vi "GetSensorValues.vi"(1 "Ref_BuiltInAccelerometer":T8={"DevStatus"={"status"=FALSE, "code"=0, "source"=""}, "Scaling"={"Gain (VoltsPerG)"=0.0, "Center Voltage"=0.0}, "Analog Channels"={"X-Axis"=enum."Invalid", "Y-Axis"=enum."Invalid", "Z-Axis"=enum."Invalid"}, "I2C Bus"=enum."Invalid", "SPI Bus"=enum."Invalid", "Accel Range"=0, "ADXL Axes"={"X-Axis"=FALSE, "Y-Axis"=FALSE, "Z-Axis"=FALSE}, "Handle"=0, "Device Address"=0, "Accel Type"=enum."Analog"} {"Device Address" format="%.0x"; "Accel Range" items=["+/- 2 g", "+/- 4 g", "+/- 8 g", "+/- 16 g"]}, 3 "Rear Prox Sensor":T6, 4 "Right Prox Sensor":T6, 5 "Left Prox Sensor":T6, 6 "Upper Pressure Transducer":T6, 8 "Ref_Compressor":T15, 9 "Front-Right Prox Sensor":T6, 10 "Ref_ElevatorEncoder":T1={"DeviceStatus"={"status"=FALSE, "code"=0, "source"=""}, "Type"=enum."PWM", "PWM"={"PWM Channel"=enum."Invalid", "DeadBand"={"Name"="", "maxPositivePwm"=0, "minPositivePwm"=0, "centerPwm"=0, "maxNegativePwm"=0, "minNegativePwm"=0, "angularRange"=0}}, "CAN"={"Device Number"=0, "SetOutput VI Ref"=variant, "GetOutput VI Ref"=variant, "Enable VI Ref"=variant, "Disable VI Ref"=variant, "Data"=variant}, "Invert"=FALSE, "DIO PWM"={"PWM \"Enable\" Channel"=enum."Invalid", "DIOChannel"=enum."Invalid", "PWM Rate"=0.0}}, 11 "Front-Left Prox Sensor":T6, 12 "Ref_ElevatorLimitSwitches":T1={"DeviceStatus"={"status"=FALSE, "code"=0, "source"=""}, "Type"=enum."PWM", "PWM"={"PWM Channel"=enum."Invalid", "DeadBand"={"Name"="", "maxPositivePwm"=0, "minPositivePwm"=0, "centerPwm"=0, "maxNegativePwm"=0, "minNegativePwm"=0, "angularRange"=0}}, "CAN"={"Device Number"=0, "SetOutput VI Ref"=variant, "GetOutput VI Ref"=variant, "Enable VI Ref"=variant, "Disable VI Ref"=variant, "Data"=variant}, "Invert"=FALSE, "DIO PWM"={"PWM \"Enable\" Channel"=enum."Invalid", "DIOChannel"=enum."Invalid", "PWM Rate"=0.0}}, 15 "Tank Pressure Transducer":T6, 19 "Ground Prox Sensor":T6, 20 "Ref_Drive 1R":T1, 21 "Ref_Drive 2R":T1, 22 "Ref_Drive 3L":T1, 23 "Ref_Drive 4L":T1, 24 "Ref_Drive 5L":T1, 26 "Ref_Drive 6R":T1) -> ()   [LabVIEW 2018]
uses:
  <vilib>/Rock Robotics/WPI/AnalogChannel/WPI_AnalogChannelDevRef.ctl
  <vilib>/Rock Robotics/SystemInterfaces/AI/FPGA_AIChannel.ctl
  <vilib>/Rock Robotics/WPI/Compressor/WPI_CompressorDevRef.ctl
  <vilib>/Rock Robotics/WPI/MotorControl/WPI_MotorControlDeviceRef.ctl
  <vilib>/Rock Robotics/WPI/MotorControl/WPI_MotorControlType.ctl
  <vilib>/Rock Robotics/SystemInterfaces/DIO/FPGA_DIOPWMChannel.ctl
  <vilib>/Rock Robotics/WPI/PWM/WPI_PWMDeadband.ctl
  <vilib>/Rock Robotics/SystemInterfaces/DIO/FPGA_DIOChannel.ctl
  <vilib>/Rock Robotics/WPI/Accelerometer/WPI_AccelerometerDevRef.ctl
  <vilib>/Rock Robotics/WPI/Accelerometer/WPI_AccelerometerScaling.ctl
  <vilib>/Rock Robotics/WPI/Accelerometer/WPI_AccelerometerAnalogChannels.ctl
  <vilib>/Rock Robotics/SystemInterfaces/i2clib/i2c_bus.ctl
  <vilib>/Rock Robotics/SystemInterfaces/spilib/spi_bus.ctl
  <vilib>/Rock Robotics/WPI/Accelerometer/ADXL345 Range.ctl
  <vilib>/Rock Robotics/WPI/Accelerometer/WPI_AccelerometerADXL345 Axes.ctl
  <vilib>/Rock Robotics/WPI/DriverStation/WPI_DriverStationRobotMode2.ctl
  <vilib>/Analysis/baseanly.llb/Mean (DBL).vi
  SensorReadings.vi
  RefNums_Actuators.vi
  RobotStates.vi
  Inputs_DriverStation.vi
  <vilib>/Rock Robotics/WPI/ThirdParty/Phoenix-LabVIEW/Motor Controller/Get/CTRE_Phoenix_MotorController_GetLimitSwitchStates.vi
  <vilib>/Rock Robotics/WPI/ThirdParty/Phoenix-LabVIEW/Motor Controller/Get/CTRE_Phoenix_MotorController_GetSelectedSensorData.vi
  <vilib>/gmath/NI_Gmath.lvlib
  <vilib>/Analysis/NI_AALBase.lvlib
  <vilib>/Analysis/NI_AALPro.lvlib
panel:
  out "Pressure Leak (psi/min)":dbl format="%#_3f"
  in  "Normal Elevator Std (A)":dbl=35.0
  in  "Off Ground Time (ms)":u32=100
  in  "On Ground Time (ms)":u32=1000
  in  "Ground Distance (in)":dbl=6.0
  in  "Plot Drive Encoder Data":bool
  in  "Tank Pressure Voltage Table":dbl[](array[numeric])=[0.4, 0.7, 0.9, 1.2, 1.4, 1.7, 1.9, 2.3, 2.5, 2.8, 3.0, 3.3] format="%_6g"
  in  "Tank Pressure PSI Table":dbl[](array[numeric])=[0.0, 10.0, 20.0, 30.0, 40.0, 50.0, 60.0, 70.0, 80.0, 90.0, 100.0, 115.0] format="%_6g"
  in  "LR Voltage Table":dbl[](array[numeric])=[0.43, 0.45, 0.47, 0.55, 0.6, 0.68, 0.72, 0.81, 0.86, 0.98, 1.13, 1.36, 1.53, 1.77, 1.99, 2.26, 2.52, 2.76] format="%_6g"
  in  "LR Distance Table":dbl[](array[numeric])=[150.661, 140.6, 133.7, 120.9, 110.1, 95.3, 90.1, 80.0, 73.7, 64.6, 55.9, 45.6, 40.2, 35.0, 29.6, 24.3, 19.6, 14.8] format="%_6g"
  in  "Suction Threshold (V)":dbl=0.1
  in  "SR Voltage Table":dbl[](array[numeric])=[3.15, 2.82, 2.51, 2.16, 1.92, 1.7, 1.49, 1.3, 1.12, 0.97, 0.87, 0.79, 0.72, 0.64, 0.61, 0.58, 0.52, 0.47, 0.46, 0.45, 0.43, 0.41] format="%_6g"
  in  "SR Distance Table":dbl[](array[numeric])=[4.6, 6.6, 8.3, 10.4, 12.2, 14.1, 16.5, 19.9, 23.6, 28.2, 32.6, 36.8, 40.9, 46.3, 49.9, 53.7, 58.3, 63.5, 67.5, 71.5, 75.1, 78.9] format="%_6g"
  out "Drive Encoder Velocities":cluster{dbl, dbl}(graph)
  # "*** Alpha was set to 6 inches ***"
  # "*** Beta was set to 12 inches ***"
  # "ADXL"
  # "Analog"
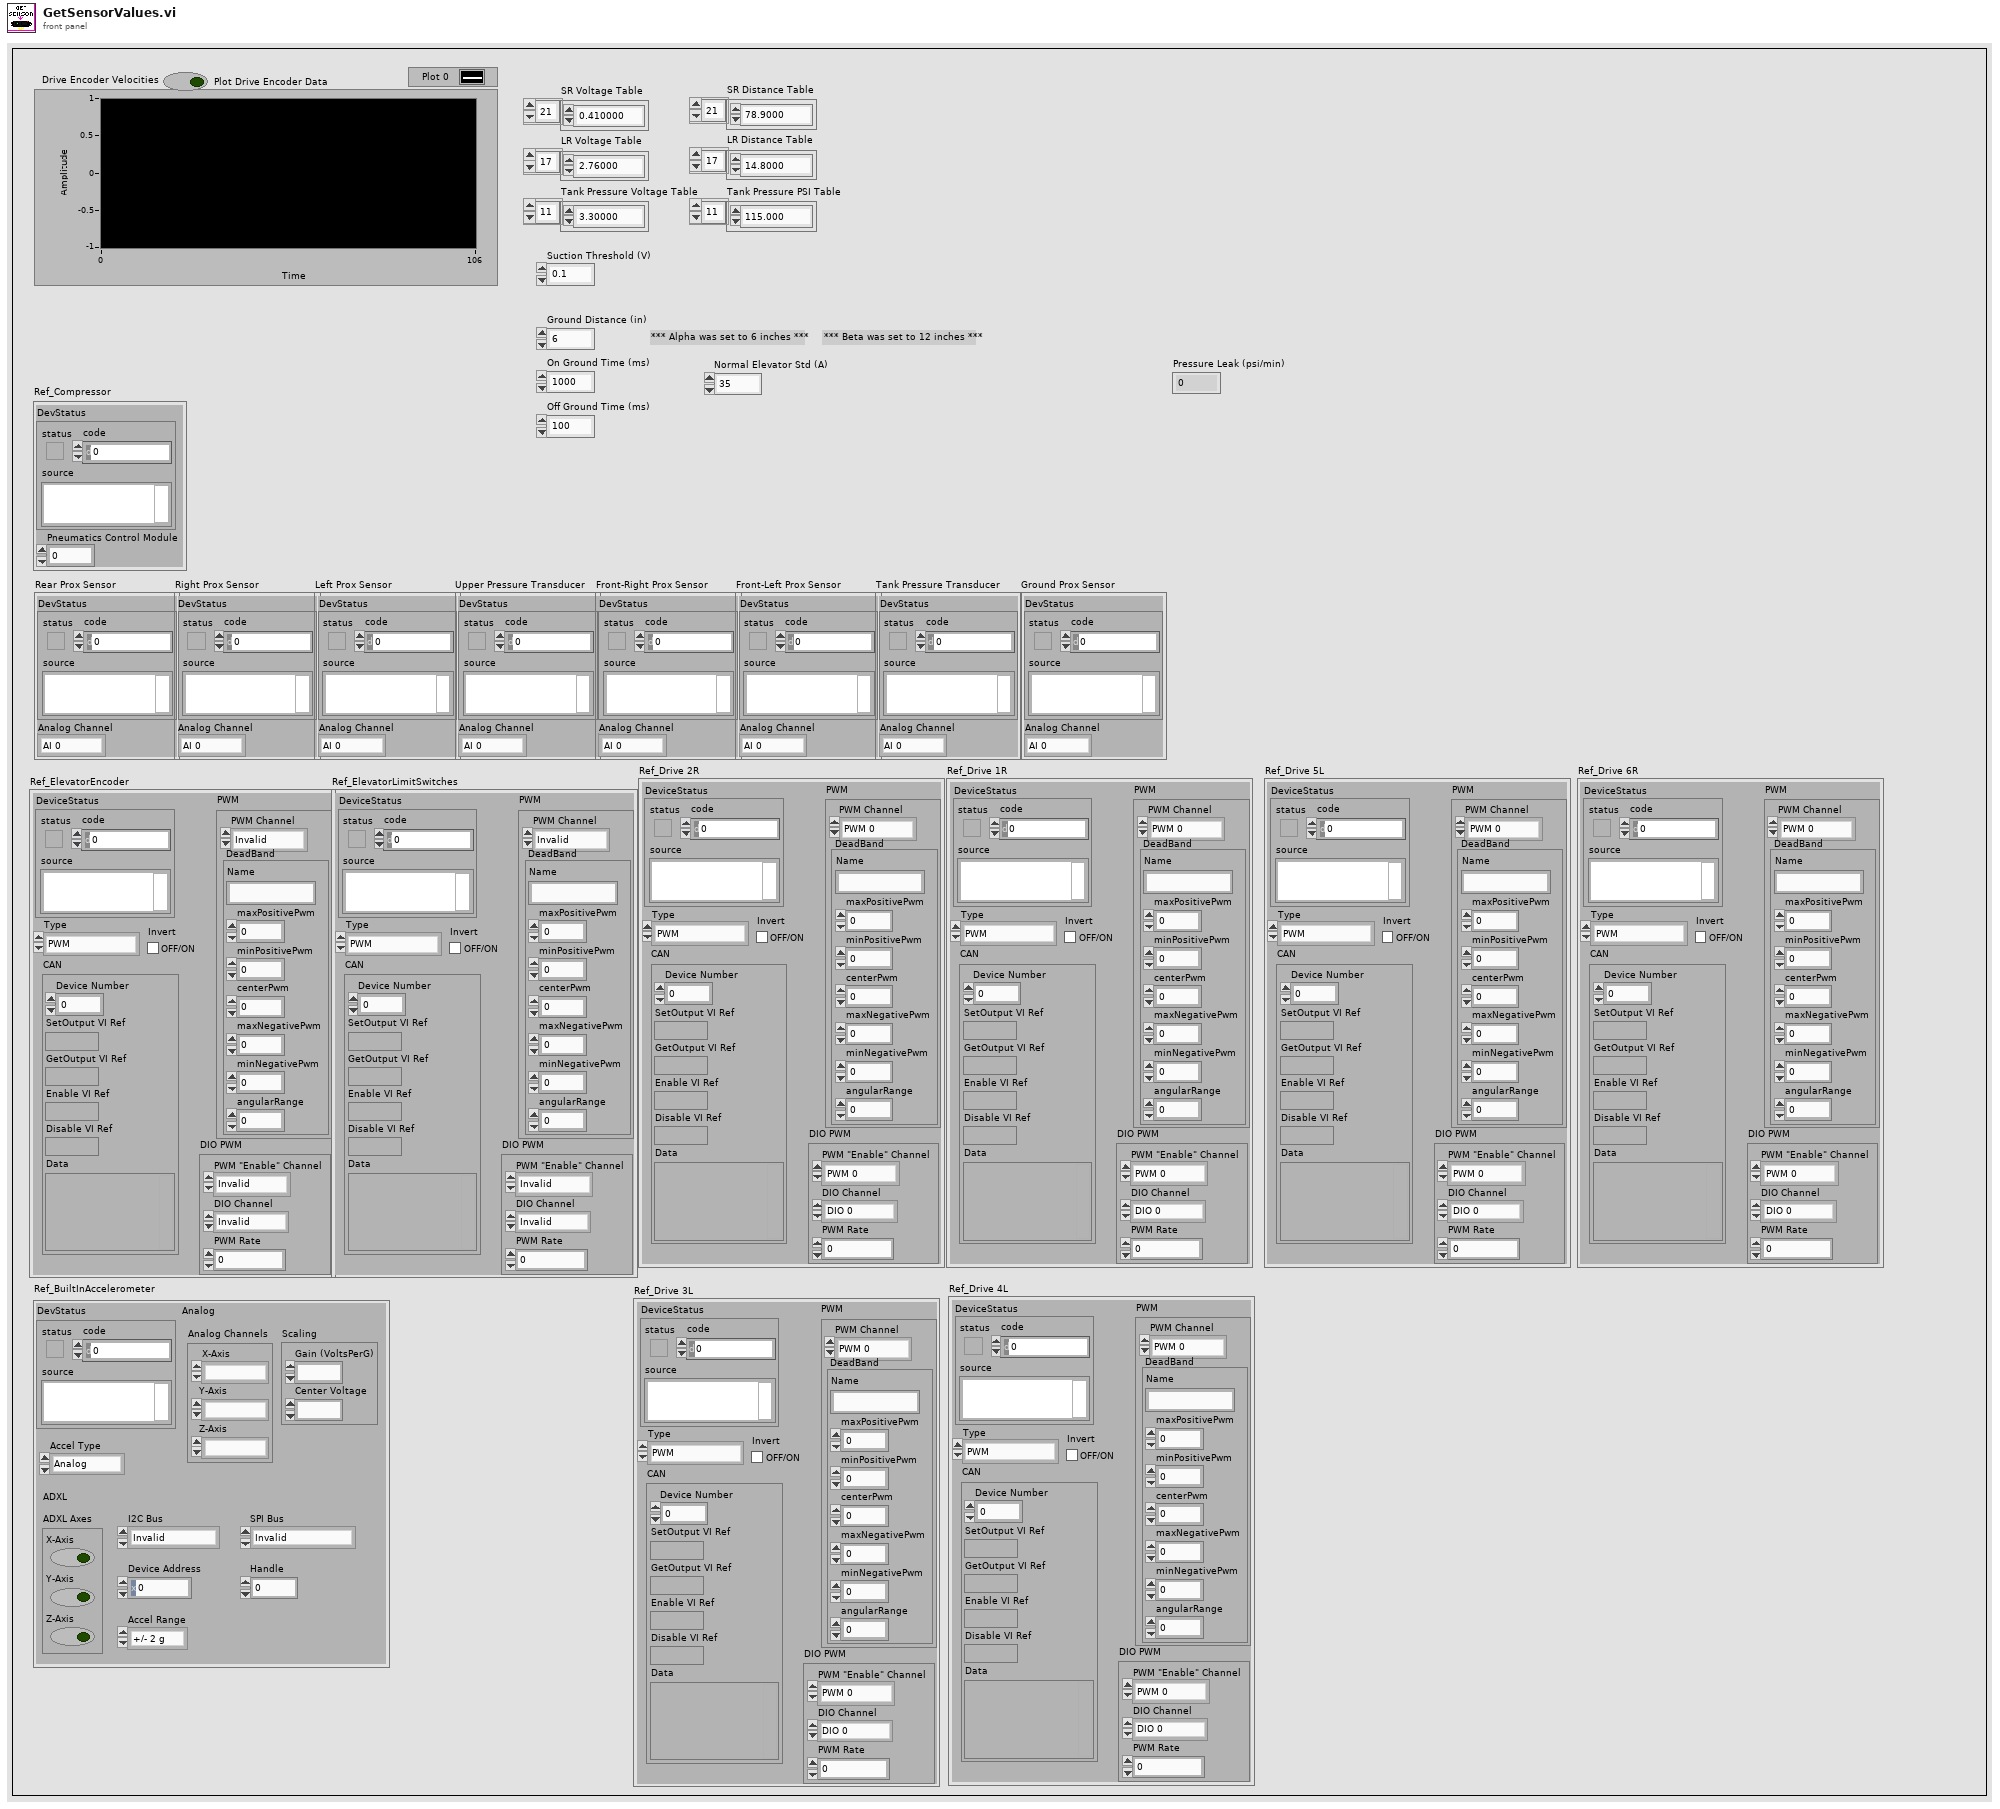
[diagram p1: front panel]
types:
  T1 = typedef "WPI_MotorControlDeviceRef.ctl" = cluster{"DeviceStatus":errorcluster, "Type":T2, "PWM":cluster{"PWM Channel":T3, "DeadBand":T4}, "CAN":cluster{"Device Number":u8, "SetOutput VI Ref":variant, "GetOutput VI Ref":variant, "Enable VI Ref":variant, "Disable VI Ref":variant, "Data":variant}, "Invert":bool, "DIO PWM":cluster{"PWM \"Enable\" Channel":T3, "DIOChannel":T5, "PWM Rate":dbl}}
  T2 = typedef "WPI_MotorControlType.ctl" = enum16{"PWM", "CAN", "DIO PWM"}
  T3 = typedef "FPGA_DIOPWMChannel.ctl" = enum8{"PWM 0", "PWM 1", "PWM 2", "PWM 3", "PWM 4", "PWM 5", "PWM 6", "PWM 7", "PWM 8", "PWM 9", "PWM MXP 0", "PWM MXP 1", "PWM MXP 2", "PWM MXP 3", "PWM MXP 4", "PWM MXP 5", "PWM MXP 6", "PWM MXP 7", "PWM MXP 8", "PWM MXP 9", "Invalid"}
  T4 = typedef "WPI_PWMDeadband.ctl" = cluster{"Name":string, "maxPositivePwm":i32, "minPositivePwm":i32, "centerPwm":i32, "maxNegativePwm":i32, "minNegativePwm":i32, "angularRange":u16}
  T5 = typedef "FPGA_DIOChannel.ctl" = enum8{"DIO 0", "DIO 1", "DIO 2", "DIO 3", "DIO 4", "DIO 5", "DIO 6", "DIO 7", "DIO 8", "DIO 9", "DIO MXP 0", "DIO MXP 1", "DIO MXP 2", "DIO MXP 3", "DIO MXP 4", "DIO MXP 5", "DIO MXP 6", "DIO MXP 7", "DIO MXP 8", "DIO MXP 9", "DIO MXP 10", "DIO MXP 11", "DIO MXP 12", "DIO MXP 13", "DIO MXP 14", "DIO MXP 15", "SPI Port CS1", "SPI Port CS2", "SPI Port CS3", "SPI Port MISO", "SPI Port MOSI", "Invalid"}
  T6 = typedef "WPI_AnalogChannelDevRef.ctl" = cluster{"DevStatus":errorcluster, "Analog Channel":T7}
  T7 = typedef "FPGA_AIChannel.ctl" = enum8{"AI 0", "AI 1", "AI 2", "AI 3", "AI MXP 0", "AI MXP 1", "AI MXP 2", "AI MXP 3", "Invalid"}
  T8 = typedef "WPI_AccelerometerDevRef.ctl" = cluster{"DevStatus":errorcluster, "Scaling":T9, "Analog Channels":T10, "I2C Bus":T11, "SPI Bus":T12, "Accel Range":T13, "ADXL Axes":T14, "Handle":i32, "Device Address":u8, "Accel Type":enum16{"Analog", "ADXL345 I2C", "ADXL345 SPI", "Internal", "ADXL362 SPI"}}
  T9 = typedef "WPI_AccelerometerScaling.ctl" = cluster{"Gain (VoltsPerG)":dbl, "Center Voltage":dbl}
  T10 = typedef "WPI_AccelerometerAnalogChannels.ctl" = cluster{"X-Axis":T7, "Y-Axis":T7, "Z-Axis":T7}
  T11 = typedef "i2c_bus.ctl" = enum16{"I2C On-Board", "I2C MXP", "Invalid"}
  T12 = typedef "spi_bus.ctl" = enum16{"SPI On-Board, CS0", "SPI On-Board, CS1", "SPI On-Board, CS2", "SPI On-Board, CS3", "SPI MXP", "Invalid"}
  T13 = typedef "ADXL345 Range.ctl" = u8
  T14 = typedef "WPI_AccelerometerADXL345 Axes.ctl" = cluster{"X-Axis":bool, "Y-Axis":bool, "Z-Axis":bool}
  T15 = typedef "WPI_CompressorDevRef.ctl" = cluster{"DevStatus":errorcluster, "Pneumatics Control Module":u8}
  T16 = typedef "WPI_DriverStationRobotMode2.ctl" = enum16{"Autonomous Disabled", "Autonomous Enabled", "Teleop Disabled", "Teleop Enabled", "Disconnected", "Finish", "Test Disabled", "Test Enabled", "Emergency Stopped"}
  T17 = cluster{"X-Axis":dbl, "Y-Axis":dbl, "Z-Axis":dbl}
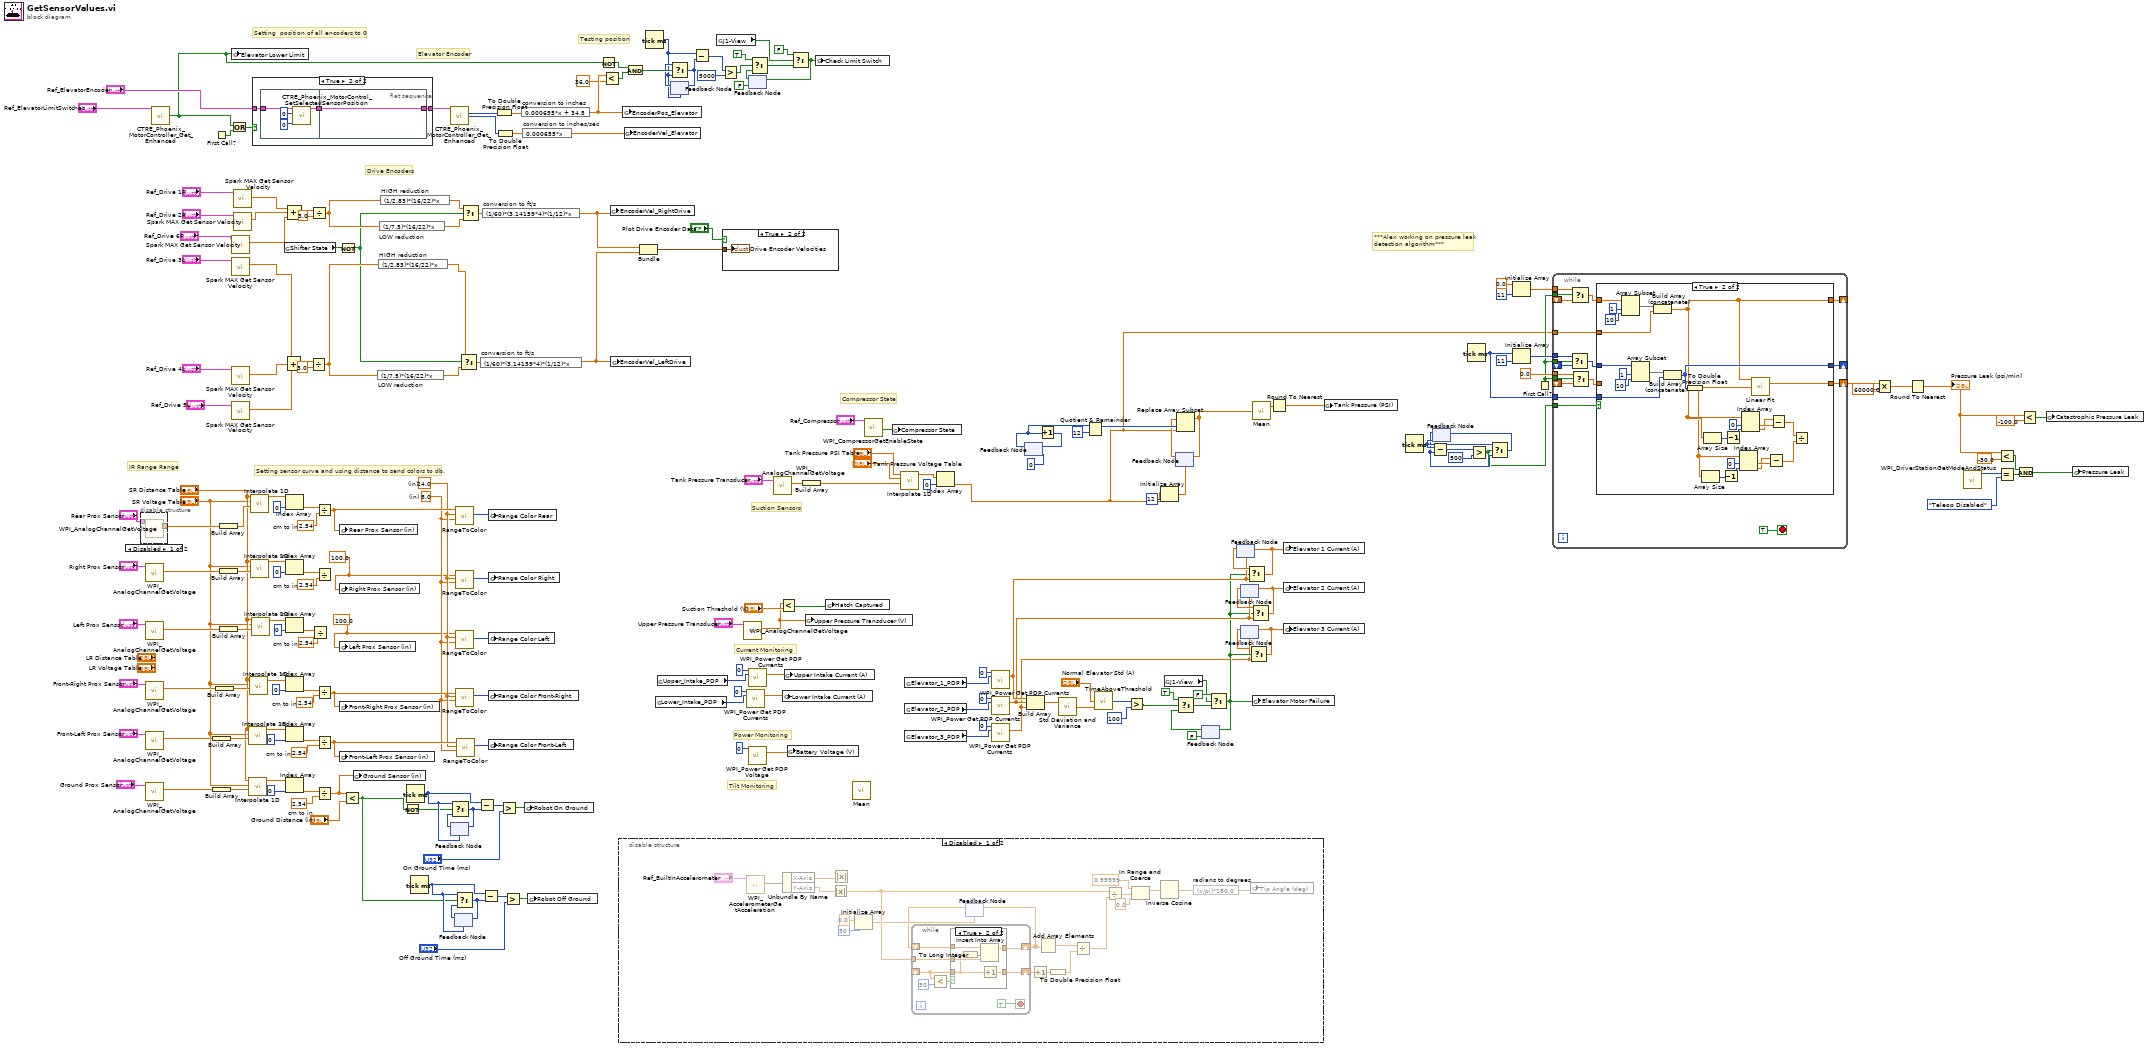
[diagram p0: block diagram]
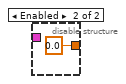
[diagram p3: hidden frame]
diagram:
  w50 = 100.0
  w51 = 100.0
  w121 = 2.54  # cm to in
  w177 = 2.54  # cm to in
  w170 = 8.0  # (in)
  w171 = 24.0  # (in)
  w194 = 2.54  # cm to in
  w200 = 2.54  # cm to in
  w207 = 2.54  # cm to in
  w214 = 2.54  # cm to in
  # "***Alex working on pressure leak\ndetection algorithm***"
  # "Elevator Encoder"
  # "Tilt Monitoring"
  # "Drive Encoders"
  # "Power Monitoring"
  # "Testing position"
  # "Setting  position of all encoders to 0"
  # "Setting sensor curve and using distance to send colors to db."
  # "Current Monitoring"
  # "Suction Sensors"
  # "Compressor State"
  # "IR Range Range"
  n1 = disable-structure shown="Disabled" {
    disable-tunnel: [w220 0.0 ("Voltage")] -> w218
    disable-tunnel: "Rear Prox Sensor" -> [w219 _]
    frame Disabled {
      n2 = call <vilib>:"WPI_AnalogChannelGetVoltage.vi"("AIDeviceRef"=w219) -> ("Voltage"=w220:dbl)  [unwired: 8 in, 2 out]
    }
    frame Enabled {
    }
  }
  n3 = call <vilib>:"WPI_AnalogChannelGetVoltage.vi"("AIDeviceRef"="Right Prox Sensor") -> ("Voltage"=w212:dbl)  [unwired: 8 in, 2 out]
  n4 = call <vilib>:"WPI_AnalogChannelGetVoltage.vi"("AIDeviceRef"="Left Prox Sensor") -> ("Voltage"=w205:dbl)  [unwired: 8 in, 2 out]
  n5 = call <vilib>:"WPI_AnalogChannelGetVoltage.vi"("AIDeviceRef"="Front-Right Prox Sensor") -> ("Voltage"=w182:dbl)  [unwired: 8 in, 2 out]
  n6 = call <vilib>:"WPI_AnalogChannelGetVoltage.vi"("AIDeviceRef"="Front-Left Prox Sensor") -> ("Voltage"=w175:dbl)  [unwired: 8 in, 2 out]
  n7 = call <vilib>:"WPI_AnalogChannelGetVoltage.vi"("AIDeviceRef"="Ground Prox Sensor") -> ("Voltage"=w120:dbl)  [unwired: 8 in, 2 out]
  n8 = call-poly <vilib>:"CTRE_Phoenix_MotorController_Get_Enhanced.vi"("PhoenixMotorControlDevRef"="Ref_ElevatorLimitSwitches") -> ("Reverse Limit Closed?"=w67:bool)  [unwired: 11 in, 3 out]
  n9 = First Call?() -> (First Call?: T/F=w125:bool)
  n10 = Build Array(w175) -> (w180:dbl[])
  n11 = Build Array(w120) -> (w124:dbl[])
  n12 = Build Array(w182) -> (w198:dbl[])
  n13 = Build Array(w218) -> (w192:dbl[])
  n14 = Build Array(w212) -> (w211:dbl[])
  n15 = Build Array(w205) -> (w204:dbl[])
  n16 = Or(x=w67, y=w125) -> (x .or. y?=w126:bool)
  n17 = global write "SensorReadings.vi" "Elevator Lower Limit"(w67) -> ()
  n18 = call <vilib>:"Spark MAX Get Sensor Velocity.vi"("MotorControlDevRef in"="Ref_Drive 6R") -> ("Sensor Velocity"=w47:dbl)  [unwired: 7 in, 3 out]
  n19 = call <vilib>:"Spark MAX Get Sensor Velocity.vi"("MotorControlDevRef in"="Ref_Drive 3L") -> ("Sensor Velocity"=w153:dbl)  [unwired: 7 in, 3 out]
  n20 = call <vilib>:"Spark MAX Get Sensor Velocity.vi"("MotorControlDevRef in"="Ref_Drive 4L") -> ("Sensor Velocity"=w152:dbl)  [unwired: 7 in, 3 out]
  n21 = call <vilib>:"Spark MAX Get Sensor Velocity.vi"("MotorControlDevRef in"="Ref_Drive 5L") -> ("Sensor Velocity"=w46:dbl)  [unwired: 7 in, 3 out]
  n22 = call <vilib>:"Spark MAX Get Sensor Velocity.vi"("MotorControlDevRef in"="Ref_Drive 1R") -> ("Sensor Velocity"=w158:dbl)  [unwired: 7 in, 3 out]
  n23 = call <vilib>:"Spark MAX Get Sensor Velocity.vi"("MotorControlDevRef in"="Ref_Drive 2R") -> ("Sensor Velocity"=w99:dbl)  [unwired: 7 in, 3 out]
  n24 = call <vilib>:"Interpolate 1D.vi"("xi"=w180, "X"="SR Voltage Table", "Y"="SR Distance Table") -> ("yi"=w174:dbl[])  [unwired: 6 in, 2 out]
  n25 = call <vilib>:"Interpolate 1D.vi"("xi"=w124, "X"="SR Voltage Table", "Y"="SR Distance Table") -> ("yi"=w119:dbl[])  [unwired: 6 in, 2 out]
  n26 = call <vilib>:"Interpolate 1D.vi"("xi"=w198, "X"="SR Voltage Table", "Y"="SR Distance Table") -> ("yi"=w195:dbl[])  [unwired: 6 in, 2 out]
  n27 = call <vilib>:"Interpolate 1D.vi"("xi"=w192, "X"="SR Voltage Table", "Y"="SR Distance Table") -> ("yi"=w215:dbl[])  [unwired: 6 in, 2 out]
  n28 = call <vilib>:"Interpolate 1D.vi"("xi"=w211, "X"="SR Voltage Table", "Y"="SR Distance Table") -> ("yi"=w208:dbl[])  [unwired: 6 in, 2 out]
  n29 = call <vilib>:"Interpolate 1D.vi"("xi"=w204, "X"="SR Voltage Table", "Y"="SR Distance Table") -> ("yi"=w201:dbl[])  [unwired: 6 in, 2 out]
  n30 = case shown="True" w126 {
    tunnel: "Ref_ElevatorEncoder" -> [w222 w225]
    tunnel: [w222 w223] -> w131
    frame False {
    }
    frame True {
      n31 = flat-sequence {
        tunnel: w225 -> [w229]
        tunnel: [w228] -> w224
        tunnel: [w230] -> w223
        tunnel: w224 -> [w230]
        frame #0 {
          n32 = call <vilib>:"CTRE_Phoenix_MotorControl_SetSelectedSensorPosition.vi"("pidLoopIdx"=u32 0, "New Sensor Position"=0, "PhoenixMotorControlDevRef"=w229) -> ("PhoenixMotorControlDevRef"=w228:T1)  [unwired: 7 in, 1 out]
        }
        frame #1 {
        }
      }
    }
  }
  n33 = global read "RobotStates.vi" "Shifter State"() -> (w145:bool)
  n34 = Index Array(array=w215, index=0) -> (element=w216:dbl)
  n35 = Index Array(array=w208, index=0) -> (element=w209:dbl)
  n36 = Index Array(array=w201, index=0) -> (element=w202:dbl)
  n37 = Index Array(array=w195, index=0) -> (element=w196:dbl)
  n38 = Index Array(array=w174, index=0) -> (element=w178:dbl)
  n39 = Index Array(array=w119, index=0) -> (element=w122:dbl)
  n40 = Compound Arithmetic op=ADD(w153, w152, w46) -> (w155:dbl)
  n41 = Compound Arithmetic op=ADD(w158, w99, w47) -> (w157:dbl)
  n42 = Divide(x=w155, y=3.0) -> (x/y=w146:dbl)
  n43 = Divide(x=w157, y=3.0) -> (x/y=w149:dbl)
  n44 = Divide(x=w202, y=w200) -> ()  [unwired: 1 out]
  n45 = Divide(x=w216, y=w214) -> (x/y=w191:dbl)
  n46 = Divide(x=w209, y=w207) -> ()  [unwired: 1 out]
  n47 = Divide(x=w196, y=w194) -> (x/y=w190:dbl)
  n48 = Divide(x=w178, y=w177) -> (x/y=w176:dbl)
  n49 = Divide(x=w122, y=w121) -> (x/y=w102:dbl)
  n50 = Not(x=w145) -> (.not. x?=w133:bool)
  n51 = global write "SensorReadings.vi" "Rear Prox Sensor (in)"(w191) -> ()
  n52 = global write "SensorReadings.vi" "Right Prox Sensor (in)"(w51) -> ()
  n53 = global write "SensorReadings.vi" "Left Prox Sensor (in)"(w50) -> ()
  n54 = global write "SensorReadings.vi" "Front-Right Prox Sensor (in)"(w190) -> ()
  n55 = global write "SensorReadings.vi" "Front-Left Prox Sensor (in)"(w176) -> ()
  n56 = Less?(x=w102, y="Ground Distance (in)") -> (x < y?=w101:bool)
  n57 = global write "SensorReadings.vi" "Ground Sensor (in)"(w102) -> ()
  n58 = expression code="(1/7.5)*(16/22)*x" "LOW reduction"(w146) -> (w147:dbl)
  n59 = expression code="(1/2.83)*(16/22)*x" "HIGH reduction"(w146) -> (w148:dbl)
  n60 = expression code="(1/7.5)*(16/22)*x" "LOW reduction"(w149) -> (w150:dbl)
  n61 = expression code="(1/2.83)*(16/22)*x" "HIGH reduction"(w149) -> (w151:dbl)
  n62 = Not(x=w101) -> (.not. x?=w100:bool)
  n63 = Tick Count (ms)() -> (millisecond timer value=w112:u32)
  n64 = Tick Count (ms)() -> (millisecond timer value=w107:u32)
  n65 = feedback #1(w112) -> (w114:u32)
  n66 = call-poly <vilib>:"CTRE_Phoenix_MotorController_Get_Enhanced.vi"("PhoenixMotorControlDevRef"=w131) -> ("Position (Raw Sensor Units)"=w130:i32, "Velocity (Raw Sensor Units per 100 ms)"=w128:i32)  [unwired: 11 in, 2 out]
  n67 = Select(t=w112, s=w100, f=w114) -> (s? t:f=w113:u32)
  n68 = feedback-in #1(w113) -> ()
  n69 = feedback #2(w107) -> (w109:u32)
  n70 = call "RangeToColor.vi"("Really Close (in)"=w170, "Close (in)"=w171, "Range (in)"=w191) -> ("Range Color"=w189:u32)  [unwired: 8 in]
  n71 = call "RangeToColor.vi"("Really Close (in)"=w170, "Close (in)"=w171, "Range (in)"=w51) -> ("Range Color"=w188:u32)  [unwired: 8 in]
  n72 = call "RangeToColor.vi"("Really Close (in)"=w170, "Close (in)"=w171, "Range (in)"=w50) -> ("Range Color"=w187:u32)  [unwired: 8 in]
  n73 = call "RangeToColor.vi"("Really Close (in)"=w170, "Close (in)"=w171, "Range (in)"=w190) -> ("Range Color"=w186:u32)  [unwired: 8 in]
  n74 = Select(t=w107, s=w101, f=w109) -> (s? t:f=w108:u32)
  n75 = feedback-in #2(w108) -> ()
  n76 = call "RangeToColor.vi"("Really Close (in)"=w170, "Close (in)"=w171, "Range (in)"=w176) -> ("Range Color"=w172:u32)  [unwired: 8 in]
  n77 = Select(t=w148, s=w133, f=w147) -> (s? t:f=w135:dbl)
  n78 = Select(t=w151, s=w133, f=w150) -> (s? t:f=w137:dbl)
  n79 = Subtract(x=w112, y=w113) -> (x-y=w111:u32)
  n80 = expression code="(1/60)*(3.14159*4)*(1/12)*x" "conversion to ft/s"(w135) -> (w134:dbl)
  n81 = Subtract(x=w107, y=w108) -> (x-y=w106:u32)
  n82 = expression code="(1/60)*(3.14159*4)*(1/12)*x" "conversion to ft/s"(w137) -> (w136:dbl)
  n83 = global write "SensorReadings.vi" "Range Color Rear"(w189) -> ()
  n84 = global write "SensorReadings.vi" "Range Color Right"(w188) -> ()
  n85 = global write "SensorReadings.vi" "Range Color Left"(w187) -> ()
  n86 = global write "SensorReadings.vi" "Range Color Front-Right"(w186) -> ()
  n87 = global write "SensorReadings.vi" "Range Color Front-Left"(w172) -> ()
  n88 = To Double Precision Float(number=w130) -> (double precision float=w132:dbl)
  n89 = To Double Precision Float(number=w128) -> (double precision float=w129:dbl)
  n90 = Greater?(x=w111, y="On Ground Time (ms)") -> (0:w110:bool)
  n91 = Greater?(x=w106, y="Off Ground Time (ms)") -> (0:w105:bool)
  n92 = expression code="0.000655*x + 34.5" "conversion to inches"(w132) -> (w70:dbl)
  n93 = expression code="0.000655*x" "conversion to inches/sec"(w129) -> (w127:dbl)
  n94 = global write "SensorReadings.vi" "Robot On Ground"(w110) -> ()
  n95 = global write "SensorReadings.vi" "Robot Off Ground"(w105) -> ()
  n96 = Not(x=w67) -> (.not. x?=w69:bool)
  n97 = Less?(x=w70, y=36.0) -> (x < y?=w68:bool)
  n98 = global write "SensorReadings.vi" "EncoderVel_RightDrive"(w136) -> ()
  n99 = global write "SensorReadings.vi" "EncoderVel_LeftDrive"(w134) -> ()
  n100 = disable-structure shown="Disabled" {
    frame Disabled {
      n101 = call <vilib>:"WPI_AccelerometerGetAcceleration.vi"("AccelerometerDevRef"="Ref_BuiltInAccelerometer") -> ("Accelerations"=w251:T17)  [unwired: 8 in, 2 out]
      n102 = Unbundle By Name(w251) -> ("X-Axis"=w249:dbl, "Y-Axis"=w248:dbl)
      n103 = Absolute Value(x=w248) -> (abs(x)=w239:dbl)
      n104 = Absolute Value(x=w249) -> ()  [unwired: 1 out]
      n105 = Initialize Array(0.0 ("element"), 50 ("dimension size")) -> (w236:dbl[])
      n106 = feedback #3(w236) -> (w235:dbl[])
      n107 = while {
        shift-right: [w257] -> w237
        shift-left: w235 -> [w258]
        tunnel: w239 -> [w252]
        shift-right: [w256] -> w242
        shift-left: _ -> [w254]
        stop <- TRUE stop-if-true
        n108 = Less?(x=w254, y=50) -> (x < y?=w255:bool)
        n109 = case shown="True" w255 {
          tunnel: w258 -> [w261 w267]
          tunnel: [w261 w266] -> w257
          tunnel: w252 -> [_ w265]
          tunnel: w254 -> [w260 w264]
          tunnel: [w260 w263] -> w256
          frame False {
          }
          frame True {
            n110 = To Long Integer(number=w264) -> (32bit integer=w262:i32)
            n111 = Insert Into Array(array=w267, index=w262, new element=w265) -> (w266:dbl[])
            n112 = Increment(x=w264) -> (x+1=w263:dbl)
          }
        }
      }
      n113 = feedback-in #3(w237) -> ()
      n114 = Increment(x=w242) -> (x+1=w241:dbl)
      n115 = Add Array Elements(numeric array=w237) -> (sum=w243:dbl)
      n116 = To Double Precision Float(number=w241) -> (double precision float=w240:dbl)
      n117 = Divide(x=w243, y=w240) -> (x/y=w238:dbl)
      n118 = Divide(x=w239, y=w238) -> (x/y=w234:dbl)
      n119 = In Range and Coerce(upper limit=0.99999, x=w234, lower limit=0.0) -> (coerced(x)=w233:dbl)  [unwired: 1 out]
      n120 = Inverse Cosine(1:w233) -> (0:w246:dbl)
      n121 = expression code="(x/pi)*180.0" "radians to degrees"(w246) -> (w247:dbl)
      n122 = global write "SensorReadings.vi" "Tip Angle (deg)"(w247) -> ()
    }
    frame Enabled {
    }
  }
  n123 = global write "SensorReadings.vi" "EncoderPos_Elevator"(w70) -> ()
  n124 = global write "SensorReadings.vi" "EncoderVel_Elevator"(w127) -> ()
  n125 = Compound Arithmetic op=AND(w69, w68) -> (w60:bool)
  n126 = Bundle(w136, w134) -> (w144:cluster{dbl, dbl})  [unwired: 1 in]
  n127 = Tick Count (ms)() -> (millisecond timer value=w54:u32)
  n128 = global read "RefNums_Actuators.vi" "Lower_Intake_PDP"() -> (w165:i32)
  n129 = global read "RefNums_Actuators.vi" "Upper_Intake_PDP"() -> (w168:i32)
  n130 = feedback #4(w54) -> (w59:u32)
  n131 = Select(t=w59, s=w60, f=w54) -> (s? t:f=w55:u32)
  n132 = feedback-in #4(w55) -> ()
  n133 = Subtract(x=w54, y=w55) -> (x-y=w53:u32)
  n134 = global read "Inputs_DriverStation.vi" "J1-View"() -> (w61:bool)
  n135 = Greater?(x=w53, y=u32 5000) -> (0:w56:bool)
  n136 = case shown="True" "Plot Drive Encoder Data" {
    tunnel: w144 -> [_ w268]
    frame False {
    }
    frame True {
      "Drive Encoder Velocities" <- w268
    }
  }
  n137 = call <vilib>:"WPI_AnalogChannelGetVoltage.vi"("AIDeviceRef"="Upper Pressure Transducer") -> ("Voltage"=w163:dbl)  [unwired: 8 in, 2 out]
  n138 = call <vilib>:"WPI_Power Get PDP Currents.vi"("Power Distribution Panel (0)"=u8 0, "PDP Channel"=w165) -> ("current (A)"=w164:dbl)  [unwired: 11 in, 2 out]
  n139 = call <vilib>:"WPI_Power Get PDP Currents.vi"("Power Distribution Panel (0)"=u8 0, "PDP Channel"=w168) -> ("current (A)"=w167:dbl)  [unwired: 11 in, 2 out]
  n140 = call <vilib>:"WPI_Power Get PDP Voltage.vi"("Power Distribution Panel (0)"=u8 0) -> ("voltage (V)"=w161:dbl)  [unwired: 13 in, 1 out]
  n141 = feedback #5(FALSE) -> (w66:bool)
  n142 = Select(t=TRUE, s=w56, f=w66) -> (s? t:f=w63:bool)
  n143 = call <vilib>:"WPI_AnalogChannelGetVoltage.vi"("AIDeviceRef"="Tank Pressure Transducer") -> ("Voltage"=w39:dbl)  [unwired: 8 in, 2 out]
  n144 = Less?(x=w163, y="Suction Threshold (V)") -> (x < y?=w138:bool)
  n145 = global write "SensorReadings.vi" "Lower Intake Current (A)"(w164) -> ()
  n146 = global write "SensorReadings.vi" "Upper Intake Current (A)"(w167) -> ()
  n147 = global write "SensorReadings.vi" "Battery Voltage (V)"(w161) -> ()
  n148 = Select(t=FALSE, s=w61, f=w63) -> (s? t:f=w52:bool)
  n149 = feedback-in #5(w52) -> ()
  n150 = Build Array(w39) -> (w40:dbl[])
  n151 = global write "SensorReadings.vi" "Upper Pressure Transducer (V)"(w163) -> ()
  n152 = global write "RobotStates.vi" "Check Limit Switch"(w52) -> ()
  n153 = global write "SensorReadings.vi" "Hatch Captured"(w138) -> ()
  n154 = call-poly <vilib>:"Mean.vi"() -> ()  [unwired: 1 in, 2 out]
  n155 = call <vilib>:"WPI_CompressorGetEnableState.vi"("CompressorDevRef"="Ref_Compressor") -> ("Compressor Running"=w184:bool)  [unwired: 7 in, 3 out]
  n156 = global write "RobotStates.vi" "Compressor State"(w184) -> ()
  n157 = call <vilib>:"Interpolate 1D.vi"("xi"=w40, "X"="Tank Pressure Voltage Table", "Y"="Tank Pressure PSI Table") -> ("yi"=w43:dbl[])  [unwired: 6 in, 2 out]
  n158 = global read "RefNums_Actuators.vi" "Elevator_1_PDP"() -> (w97:i32)
  n159 = global read "RefNums_Actuators.vi" "Elevator_2_PDP"() -> (w95:i32)
  n160 = global read "RefNums_Actuators.vi" "Elevator_3_PDP"() -> (w93:i32)
  n161 = Index Array(array=w43, index=0) -> (element=w11:dbl)
  n162 = call <vilib>:"WPI_Power Get PDP Currents.vi"("Power Distribution Panel (0)"=u8 0, "PDP Channel"=w97) -> ("current (A)"=w79:dbl)  [unwired: 11 in, 2 out]
  n163 = call <vilib>:"WPI_Power Get PDP Currents.vi"("Power Distribution Panel (0)"=u8 0, "PDP Channel"=w95) -> ("current (A)"=w76:dbl)  [unwired: 11 in, 2 out]
  n164 = call <vilib>:"WPI_Power Get PDP Currents.vi"("Power Distribution Panel (0)"=u8 0, "PDP Channel"=w93) -> ("current (A)"=w73:dbl)  [unwired: 11 in, 2 out]
  n165 = feedback #6(0) -> (w36:i32)
  n166 = Build Array(w79, w76, w73) -> (w92:dbl[])
  n167 = Increment(x=w36) -> (x+1=w37:i32)
  n168 = feedback-in #6(w37) -> ()
  n169 = call <vilib>:"Std Deviation and Variance.vi"("X"=w92) -> ("standard deviation"=w91:dbl)  [unwired: 1 in, 2 out]
  n170 = Quotient & Remainder(x=w36, y=12) -> (x-y*floor(x/y)=w32:i32)  [unwired: 1 out]
  n171 = call "TimeAboveThreshold.vi"("Current Value"=w91, "Threshold"="Normal Elevator Std (A)") -> ("Time Above"=w89:u32)  [unwired: 3 in]
  n172 = Greater?(x=w89, y=u32 100) -> (0:w81:bool)
  n173 = Initialize Array(w11, 12) -> (w33:dbl[])
  n174 = global read "Inputs_DriverStation.vi" "J1-View"() -> (w82:bool)
  n175 = feedback #7(w33) -> (w24:dbl[])
  n176 = Replace Array Subset(array=w24, new element=w11, index=w32) -> (w31:dbl[])
  n177 = feedback-in #7(w31) -> ()
  n178 = feedback #8(FALSE) -> (w86:bool)
  n179 = Select(t=TRUE, s=w81, f=w86) -> (s? t:f=w84:bool)
  n180 = Select(t=FALSE, s=w82, f=w84) -> (s? t:f=w74:bool)
  n181 = feedback-in #8(w74) -> ()
  n182 = feedback #9(w79) -> (w80:dbl)
  n183 = feedback #10(w76) -> (w77:dbl)
  n184 = feedback #11(w73) -> (w71:dbl)
  n185 = Select(t=w80, s=w74, f=w79) -> (s? t:f=w78:dbl)
  n186 = feedback-in #9(w78) -> ()
  n187 = Select(t=w71, s=w74, f=w73) -> (s? t:f=w72:dbl)
  n188 = feedback-in #11(w72) -> ()
  n189 = Select(t=w77, s=w74, f=w76) -> (s? t:f=w75:dbl)
  n190 = feedback-in #10(w75) -> ()
  n191 = call-poly <vilib>:"Mean.vi"("X"=w31) -> ("mean"=w30:dbl)  [unwired: 1 out]
  n192 = global write "RobotStates.vi" "Elevator Motor Failure"(w74) -> ()
  n193 = Round To Nearest(number=w30) -> (nearest integer value=w10:dbl)
  n194 = global write "SensorReadings.vi" "Elevator 1 Current (A)"(w78) -> ()
  n195 = global write "SensorReadings.vi" "Elevator 2 Current (A)"(w75) -> ()
  n196 = global write "SensorReadings.vi" "Elevator 3 Current (A)"(w72) -> ()
  n197 = global write "SensorReadings.vi" "Tank Pressure (PSI)"(w10) -> ()
  n198 = Tick Count (ms)() -> (millisecond timer value=w27:u32)
  n199 = feedback #12(w27) -> (w26:u32)
  n200 = Subtract(x=w27, y=w26) -> (x-y=w29:u32)
  n201 = Tick Count (ms)() -> (millisecond timer value=w20:u32)
  n202 = Greater?(x=w29, y=u32 500) -> (0:w19:bool)
  n203 = Select(t=w27, s=w19, f=w26) -> (s? t:f=w25:u32)
  n204 = feedback-in #12(w25) -> ()
  n205 = Initialize Array(0.0 ("element"), 11 ("dimension size")) -> (w15:dbl[])
  n206 = Initialize Array(w20, 11 ("dimension size")) -> (w14:u32[])
  n207 = First Call?() -> (First Call?: T/F=w12:bool)
  n208 = while {
    shift-right: [w283] -> _
    shift-left: _ -> [w279]
    tunnel: w11 -> [w286]
    shift-right: [w284] -> _
    shift-left: _ -> [w278]
    tunnel: w20 -> [w285]
    tunnel: w19 -> [w269]
    shift-right: [w282] -> w18
    shift-left: _ -> [w275]
    tunnel: w15 -> [w280]
    tunnel: w14 -> [w276]
    tunnel: 0.0 ("slope") -> [w273]
    tunnel: w12 -> [w272]
    tunnel: w12 -> [w271]
    tunnel: w12 -> [w270]
    stop <- TRUE stop-if-true
    n209 = Select(t=w276, s=w271, f=w278) -> (s? t:f=w277:u32[])
    n210 = Select(t=w280, s=w270, f=w279) -> (s? t:f=w281:dbl[])
    n211 = Select(t=w273, s=w272, f=w275) -> (s? t:f=w274:dbl)
    n212 = case shown="True" w269 {
      tunnel: w286 -> [_ w316]
      tunnel: w281 -> [w288 w315]
      tunnel: w277 -> [w289 w308]
      tunnel: w285 -> [_ w307]
      tunnel: [w289 w306] -> w284
      tunnel: [w288 w302] -> w283
      tunnel: [w290 w291] -> w282
      tunnel: w274 -> [w290 _]
      frame False {
      }
      frame True {
        n213 = Array Subset(array=w315, index=1, length=10) -> (w312:dbl[])
        n214 = Array Subset(array=w308, index=1, length=10) -> (w309:u32[])
        n215 = Build Array (concatenate)(w312, w316) -> (w302:dbl[])
        n216 = Build Array (concatenate)(w309, w307) -> (w306:u32[])
        n217 = To Double Precision Float(number=w306) -> (double precision float=w294:dbl[])
        n218 = Array Size(array=w294) -> (size(s)=w298:i32)
        n219 = Array Size(array=w302) -> (size(s)=w304:i32)
        n220 = Decrement(x=w298) -> (x-1=w297:i32)
        n221 = Decrement(x=w304) -> (x-1=w303:i32)
        n222 = Index Array(array=w294, index #1=0 ("index"), index #2=w297) -> (element #1=w296:dbl, element #2=w295:dbl)
        n223 = Index Array(array=w302, index #1=0 ("index"), index #2=w303) -> (element #1=w301:dbl, element #2=w300:dbl)
        n224 = call <vilib>:"Linear Fit.vi"("Y"=w302, "X"=w294) -> ("slope"=w291:dbl)  [unwired: 9 in, 4 out]
        n225 = Subtract(x=w295, y=w296) -> (x-y=w292:dbl)
        n226 = Subtract(x=w300, y=w301) -> (x-y=w293:dbl)
        n227 = Divide(x=w293, y=w292) -> ()  [unwired: 1 out]
      }
    }
  }
  n228 = Multiply(x=w18, y=60000.0) -> (x*y=w17:dbl)
  n229 = Round To Nearest(number=w17) -> (nearest integer value=w5:dbl)
  "Pressure Leak (psi/min)" <- w5
  n230 = call <vilib>:"WPI_DriverStationGetModeAndStatus.vi"() -> ("Robot Mode"=w9:T16)  [unwired: 10 in, 1 out]
  n231 = Less?(x=w5, y=-30.0) -> (x < y?=w4:bool)
  n232 = Equal?(x=w9, y=WPI_DriverStationRobotMode2."Teleop Disabled") -> (x = y?=w3:bool)
  n233 = And(x=w4, y=w3) -> (x .and. y?=w2:bool)
  n234 = Less?(x=w5, y=-100.0) -> (x < y?=w1:bool)
  n235 = global write "SensorReadings.vi" "Catastrophic Pressure Leak"(w1) -> ()
  n236 = global write "SensorReadings.vi" "Pressure Leak"(w2) -> ()
